vi "Dashboard Main.vi"() -> ()   [LabVIEW 2016]
uses:
  <vilib>/Rock Robotics/Network Tables/NT Read Numeric Array.vi
  <vilib>/Rock Robotics/Network Tables/NT Read Number.vi
  <vilib>/Rock Robotics/Network Tables/NT Write Number.vi
  <vilib>/Rock Robotics/Network Tables/NT Read Boolean.vi
panel:
  out "Camera Info":cluster{"Mbps LED":bool, "Mbps":dbl, "fps":dbl} {"fps" format="%#.1g"; "Mbps" format="%#.1g"}
  in  "Camera Settings":T1={"Frame Rate"=30, "Compression"=30, "Size"=1, "DB Camera Config"=FALSE} {"Frame Rate" scale=1.0..30.0; "Compression" scale=100.0..-1.0; "Size" items=["640x480", "320x240", "160x120"]}
  in  "TCP":refnum<k5>
  out "Robot IP":string
  in  "Dashboard Tab":T2(tab)
  in  "Select Auto":string(combo)
  out "NT Connection":bool
  out "MotorChart R":cluster{"Numeric":dbl, "Numeric":dbl}(graph)
  out "MotorChart L":cluster{"Numeric":dbl, "Numeric":dbl}(graph)
  out "MotorSliders R":cluster{"MotorSlide1":dbl, "MotorSlide2":dbl} {"MotorSlide2" scale=-1.0..1.0 scale format="%#_2e"; "MotorSlide1" scale=-1.0..1.0 scale format="%#_2e"}
  out "MotorSliders L":cluster{"MotorSlide1":dbl, "MotorSlide2":dbl} {"MotorSlide2" scale=-1.0..1.0 scale format="%#_2e"; "MotorSlide1" scale=-1.0..1.0 scale format="%#_2e"}
  out "JS1 Z":dbl(slide) scale=-1.0..1.0 scale format="%#_2e"
  out "JS1 Graph":cluster{"X":dbl, "Y":dbl}[](graph)
  out "JS1 Buttons":T3
  out "JS2 Z":dbl(slide) scale=-1.0..1.0 scale format="%#_2e"
  out "JS2 Graph":cluster{"X":dbl, "Y":dbl}[](graph)
  out "JS2 Buttons":T3
  out "Mode":T4(ring)=enum."Auto Disabled"
  in  "flywheelTarget":dbl
  out "Flywheel PID Graph":cluster{"Numeric":dbl, "Numeric":dbl}(graph)
  in  "flywheelF":dbl
  in  "flywheelD":dbl
  in  "flywheelI":dbl
  in  "flywheelP":dbl
  out "Drive PID Graph":cluster{"Numeric":dbl, "Numeric":dbl}(graph)
  in  "driveD":dbl
  in  "driveI":dbl
  in  "driveP":dbl
  out "gyroOnTarget":bool
  out "Gyro Exists":bool
  out "Gyro Heading PID":cluster{dbl, dbl}(knob) scale=-180.0..180.0
  in  "gyroD":dbl
  in  "gyroI":dbl
  in  "gyroP":dbl
  out "Tree":string(tree)
  out "Camera Image":T5(plugin-control)
  out "Background":bool
  in  "Camera Name":string(combo)="No Camera Selection"
  # "HW"
  # "Joysticks"
  # "Drive Motors"
  # "Front"
  # "Right"
  # "Left"
  # "Back"
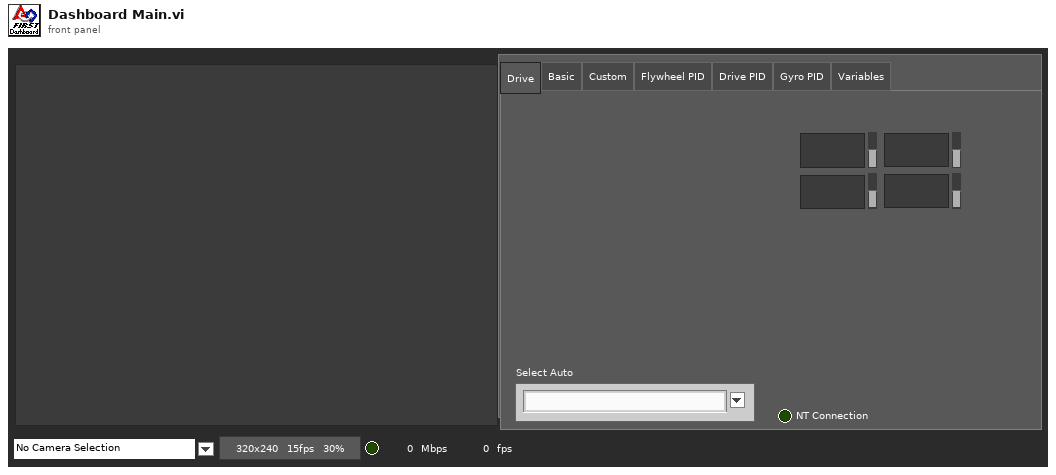
[diagram p1: front panel]
types:
  T1 = cluster{"Frame Rate":i32, "Compression":i32, "Size":u16, "DB Camera Config":bool}
  T2 = enum32{"Drive", "Basic", "Custom", "Flywheel PID", "Drive PID", "Gyro PID", "Variables"}
  T3 = cluster{bool, bool, bool, bool, bool, bool, bool, bool, bool, bool, bool, bool}
  T4 = enum8{"Tele-Op Disabled", "Tele-Op Enabled", "Auto Disabled", "Auto Enabled", "Test Disabled", "Test Enabled", "Disconnected", "No Code", "E-Stop"}
  T5 = typedef "IMAQ Image.ctl" = refnum<image>
  T6 = typedef "Image Type" = u32
  T7 = cluster{"Camera Image":refnum<vi>, "Dashboard Tab":refnum<vi>, "Background":refnum<vi>, "Tree":refnum<vi>, "Camera Settings":refnum<vi>, "Camera Name":refnum<vi>, "Camera Info":refnum<vi>}
  T8 = cluster{"Error Strings":string, "Disable Counts":cluster{u16, u16}, "Rail Faults":cluster{u16, u16, u16}, "Robot IP":string, "DB Mode":u8, "Event Info":cluster{"Name":string, "Type":u8, "Number":u16, "Replay":u8}}
  T9 = cluster{"Storage":cluster{"Disk Free":u64, "RAM Block":u32, "RAM free":u32}, "CPU Utilization":cluster{"CPU % ISR":sgl, "CPU % Time Crit":sgl, "CPU % Timed Str":sgl, "CPU % High":sgl, "CPU % Above":sgl, "CPU % Normal":sgl, "CPU % Low":sgl}, "CAN":cluster{"% Bus Utilization":sgl, "Bus Off Cnt":u32, "TX_FIFO Full Cnt":u32, "Receive Error Cnt":u8, "Transmit Error Cnt":u8}, "HID":cluster{"HID Outputs":u32, "Rumble Low":u16, "Rumble High":u16}[]}
  T10 = cluster{"Status bits":cluster{"Test Mode":bool, "Autonomous":bool, "Enabled":bool, "Code Start":bool, "Brownout":bool, "Reserved 2":bool, "Reserved 3":bool, "E-Stop":bool}, "Code Trace":cluster{"Disabled":bool, "TeleOp":bool, "Auto":bool, "Test":bool}, "Controller Type":enum16{"unknown", "cRIO", "roboRio"}, "Code?":enum16{"unknown", "noCode", "code"}, "Battery V":dbl}
  T11 = cluster{"Control Bits":cluster{"TestMode":bool, "Autonomous":bool, "Enabled":bool, "FMS Present":bool, bool, bool, bool, "E-Stop":bool}, "Team Station ":u8, "Countdown":sgl, "Joystick Values":cluster{"Axes":dbl[], "Buttons":bool[], "POVs":i16[]}[]}
  T12 = cluster{"Axes":dbl[], "Buttons":bool[], "POVs":i16[]}[]
  T13 = cluster{"Axes":dbl[], "Buttons":bool[], "POVs":i16[]}
  T14 = cluster{"Buttons[0]":bool, "Buttons[1]":bool, "Buttons[2]":bool, "Buttons[3]":bool, "Buttons[4]":bool, "Buttons[5]":bool, "Buttons[6]":bool, "Buttons[7]":bool, "Buttons[8]":bool, "Buttons[9]":bool, "Buttons[10]":bool, "Buttons[11]":bool}
  T15 = cluster{"Shift":bool, "Ctrl":bool, "Alt":bool, "Cmd":bool, "Opt":bool}
  T16 = typedef "WPI_DriverStationRobotMode2.ctl" = enum16{"Autonomous Disabled", "Autonomous Enabled", "Teleop Disabled", "Teleop Enabled", "Disconnected", "Finish", "Test Disabled", "Test Enabled", "Emergency Stopped"}
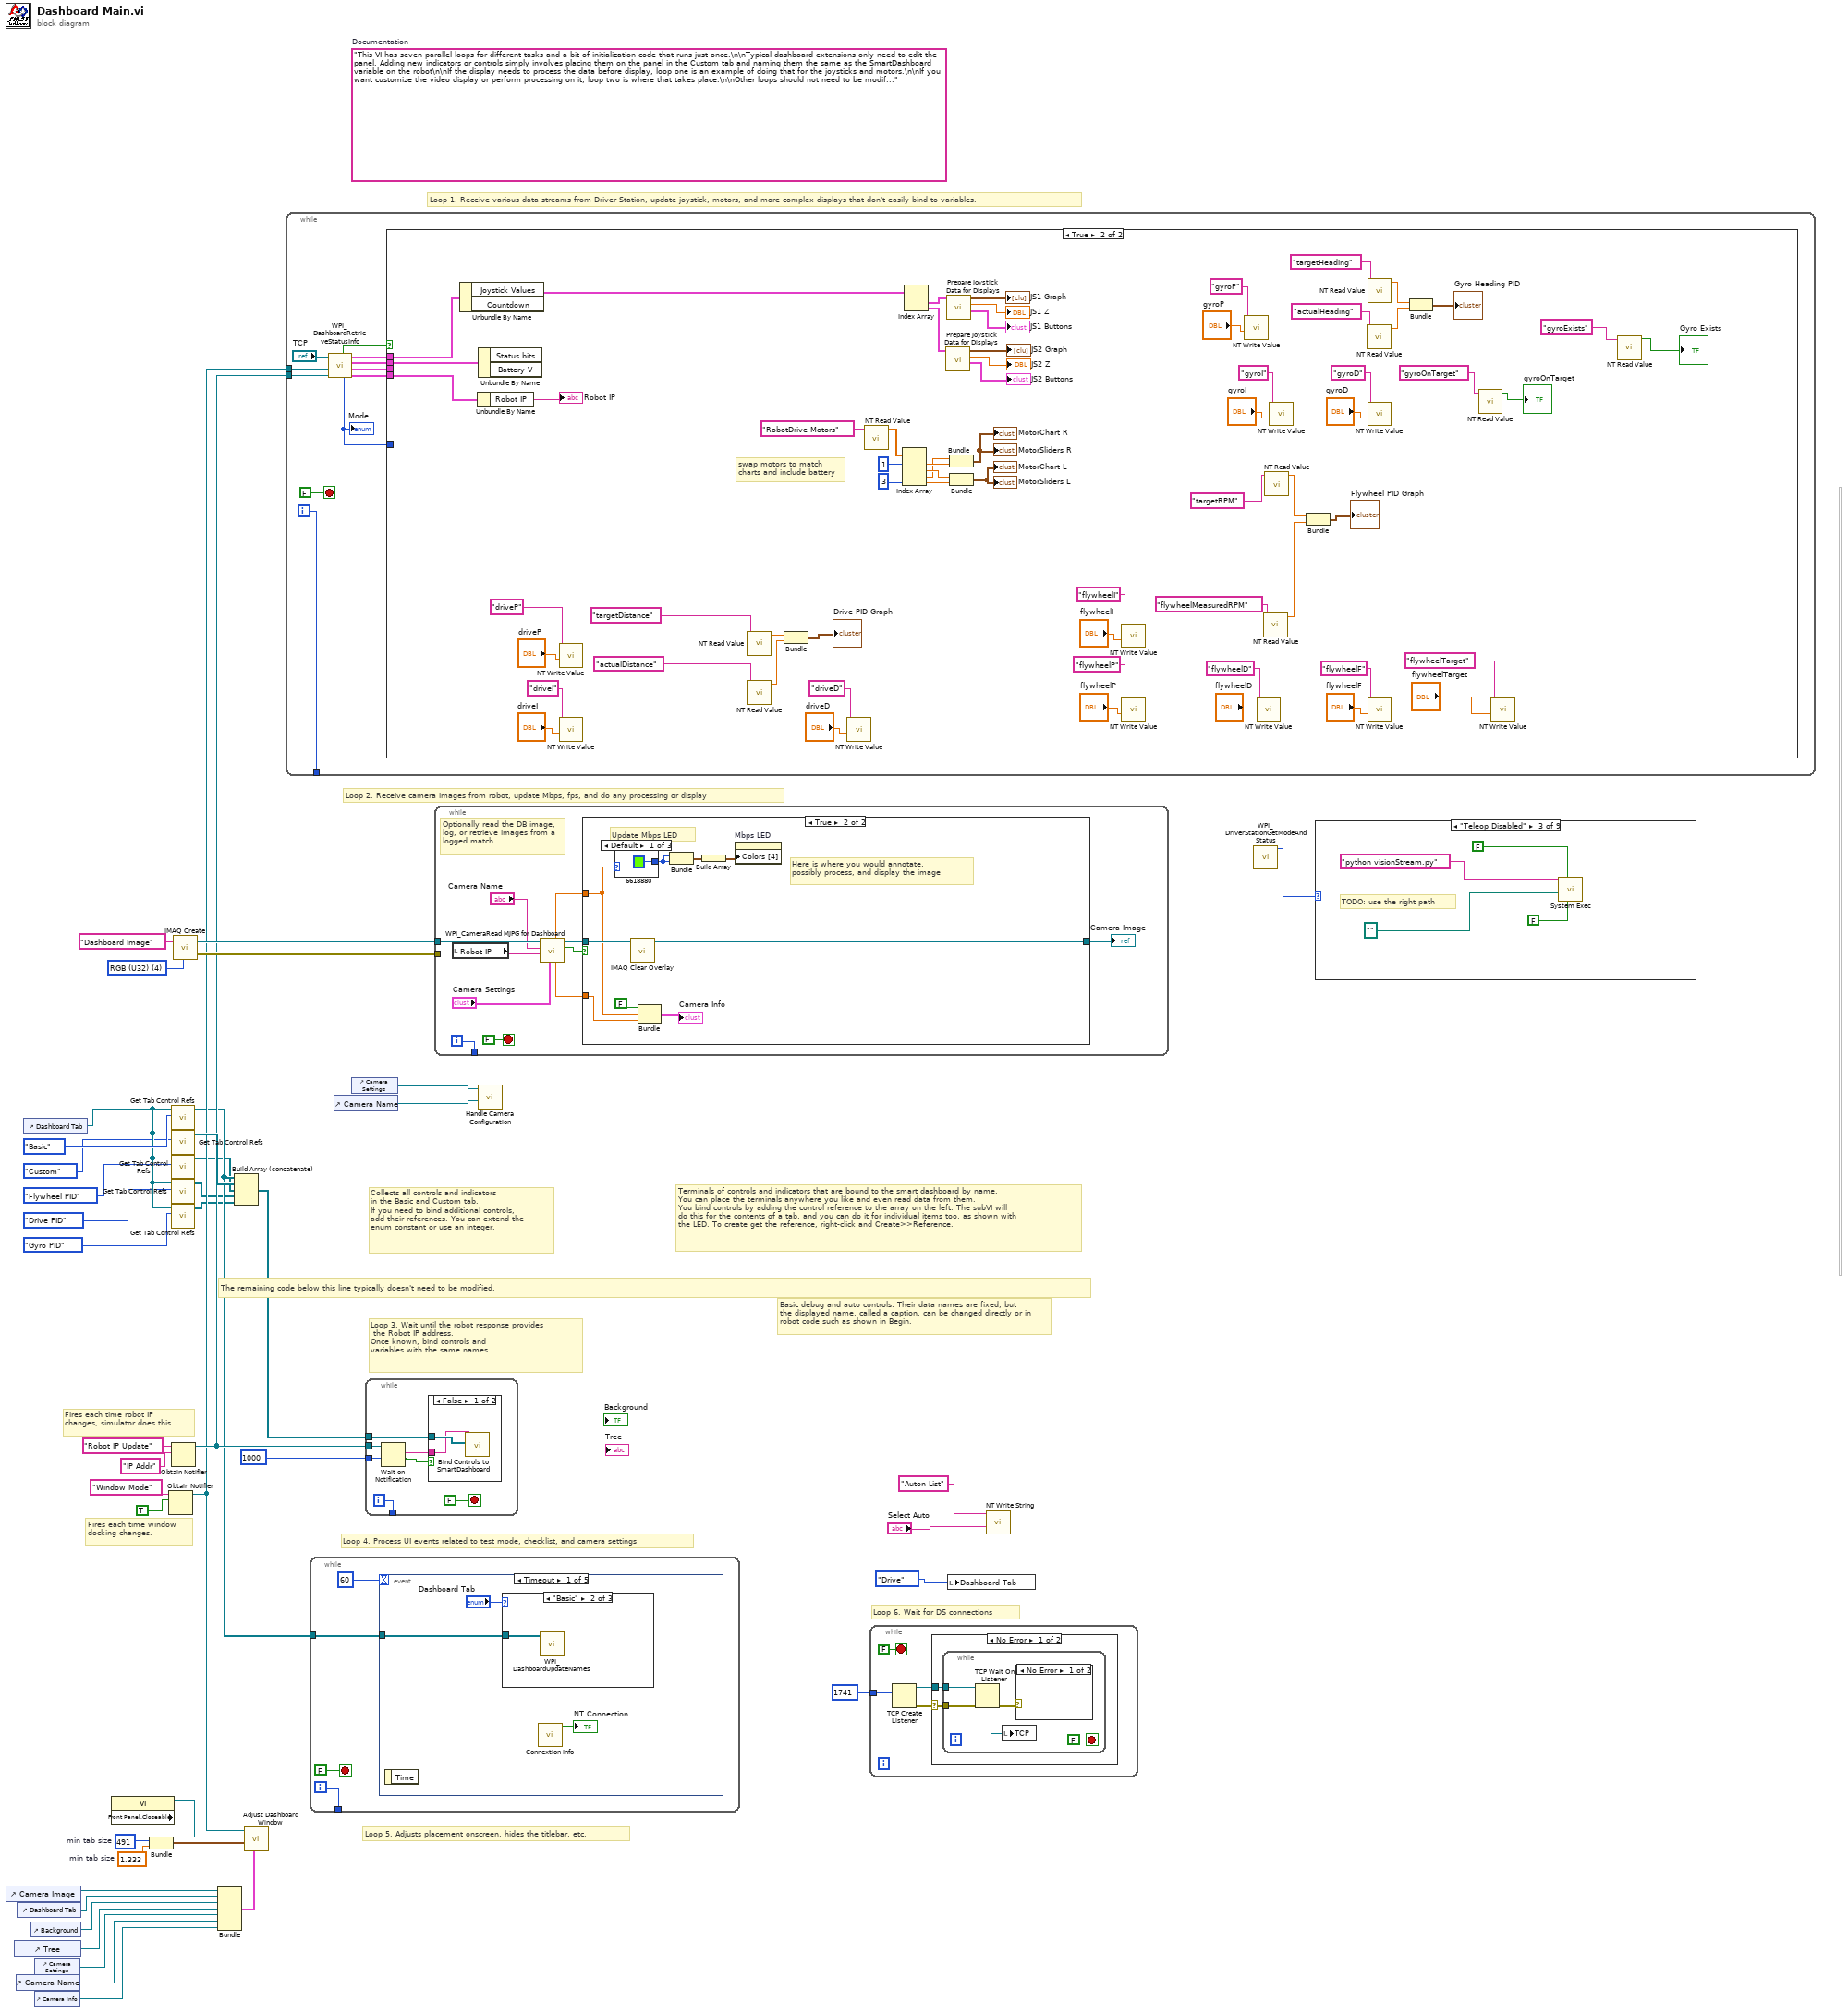
[diagram p0: block diagram]
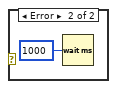
[diagram p10: hidden frame]
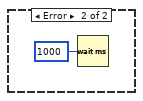
[diagram p11: hidden frame]
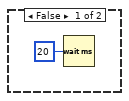
[diagram p12: hidden frame]
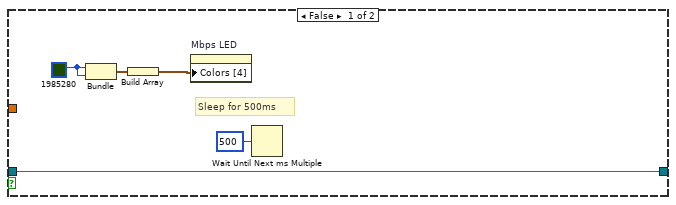
[diagram p14: hidden frame]
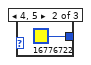
[diagram p15: hidden frame]
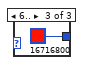
[diagram p16: hidden frame]
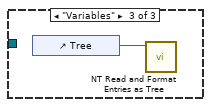
[diagram p18: hidden frame]
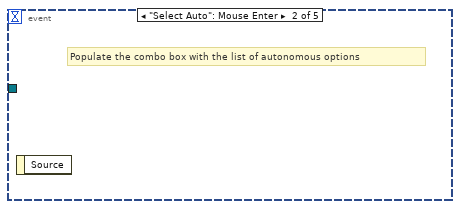
[diagram p19: hidden frame]
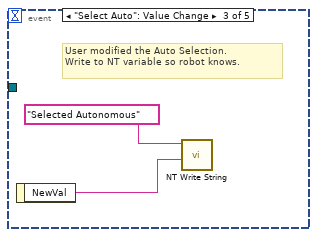
[diagram p20: hidden frame]
diagram:
  w28 = 491  # min tab size
  w27 = 1.333  # min tab size
  (unwired) "This VI has seven parallel loops for different tasks and a bit of initialization code that runs just once.\n\nTypical dashboard extensions only need to edit the panel. Adding new indicators or controls simply involves placing them on the panel in the Custom tab and naming them the same as the SmartDashboard variable on the robot\n\nIf the display needs to process the data before display, loop one is an example of doing that for the joysticks and motors.\n\nIf you want customize the video display or perform processing on it, loop two is where that takes place.\n\nOther loops should not need to be modified. They are pretty standard, and document the task they perform."  # Documentation
  w42 = T6 4 items=["Grayscale (U8)", "Grayscale (I16)", "Grayscale (SGL)", "Complex (CSG)", "RGB (U32)", "HSL (U32)", "RGB (U64)"] ("Image Type")
  # "Loop 6. Wait for DS connections"
  # "Basic debug and auto controls: Their data names are fixed, but\nthe displayed name, called a caption, can be changed directly or in\nrobot code such as shown in Begin."
  # "Fires each time robot IP\nchanges, simulator does this"
  # "Fires each time window\ndocking changes."
  # "Collects all controls and indicators\nin the Basic and Custom tab.\nIf you need to bind additional controls,\nadd their references. You can extend the\nenum constant or use an integer."
  # "The remaining code below this line typically doesn't need to be modified."
  # "Loop 4. Process UI events related to test mode, checklist, and camera settings"
  # "Terminals of controls and indicators that are bound to the smart dashboard by name.\nYou can place the terminals anywhere you like and even read data from them.\nYou bind controls by adding the control reference to the array on the left. The subVI will\ndo this for the contents of a tab, and you can do it for individual items too, as shown with\nthe LED. To create get the reference, right-click and Create>>Reference."
  # "Loop 3. Wait until the robot response provides\n the Robot IP address.\nOnce known, bind controls and\nvariables with the same names."
  # "Loop 5. Adjusts placement onscreen, hides the titlebar, etc."
  # "Loop 1. Receive various data streams from Driver Station, update joystick, motors, and more complex displays that don't easily bind to variables."
  # "Loop 2. Receive camera images from robot, update Mbps, fps, and do any processing or display"
  n1 = control-ref of="Camera Image"() -> (w30:refnum<vi>)
  n2 = control-ref of="Tree"() -> (w16:refnum<vi>)
  n3 = control-ref of="Camera Name"() -> (w14:refnum<vi>)
  n4 = control-ref of="Dashboard Tab"() -> (w29:refnum<vi>)
  n5 = control-ref of="Dashboard Tab"() -> (w8:refnum<vi>)
  n6 = control-ref of="Background"() -> (w25:refnum<vi>)
  n7 = control-ref of="Camera Settings"() -> (w15:refnum<vi>)
  n8 = control-ref of="Camera Info"() -> (w13:refnum<vi>)
  n9 = property class="VI" props=["Front Panel.Closeable"]() -> (reference out=w33:refnum<vi>)  [unwired: 2 in, 2 out]
  n10 = Bundle("min tab size"=w28, "min tab size"=w27) -> (w26:cluster{"min tab size":i32, "min tab size":dbl})  [unwired: 1 in]
  n11 = Obtain Notifier(name (unnamed)="Window Mode", notification data type=TRUE) -> (notifier out=w22:refnum<notifier>)  [unwired: 2 in, 2 out]
  n12 = call <vilib>:"Get Tab Control Refs.vi"("Page Index"=T2."Basic" ("Dashboard Tab"), "TabControl in"=w8) -> ("ControlsOnPage"=w18:refnum<vi>[])  [unwired: 9 in]
  n13 = call <vilib>:"Get Tab Control Refs.vi"("Page Index"=T2."Custom" ("Dashboard Tab"), "TabControl in"=w8) -> ("ControlsOnPage"=w32:refnum<vi>[])  [unwired: 9 in]
  n14 = call <vilib>:"Get Tab Control Refs.vi"("Page Index"=T2."Flywheel PID" ("Dashboard Tab"), "TabControl in"=w8) -> ("ControlsOnPage"=w10:refnum<vi>[])  [unwired: 9 in]
  n15 = call <vilib>:"Get Tab Control Refs.vi"("Page Index"=T2."Drive PID" ("Dashboard Tab"), "TabControl in"=w8) -> ("ControlsOnPage"=w3:refnum<vi>[])  [unwired: 9 in]
  n16 = call <vilib>:"Get Tab Control Refs.vi"("Page Index"=T2."Gyro PID" ("Dashboard Tab"), "TabControl in"=w8) -> ("ControlsOnPage"=w2:refnum<vi>[])  [unwired: 9 in]
  n17 = Obtain Notifier(name (unnamed)="Robot IP Update", notification data type="IP Addr" ("name (unnamed)")) -> (notifier out=w23:refnum<notifier>)  [unwired: 2 in, 2 out]
  n18 = call "IMAQ Create"("Image Name"="Dashboard Image", "Image Type"=w42) -> ("New Image"=w40:T5, "error out"=w39:errorcluster)  [unwired: 2 in, 1 out]
  n19 = Bundle("Camera Image"=w30, "Dashboard Tab"=w29, "Background"=w25, "Tree"=w16, "Camera Settings"=w15, "Camera Name"=w14, "Camera Info"=w13) -> (w24:T7)  [unwired: 1 in]
  n20 = Build Array (concatenate)(w18, w32, w10, w3, w2) -> (w31:refnum<vi>[])
  n21 = call "Adjust Dashboard Window.vi"("Sizing Refnums"=w24, "Size Constraints"=w26, "VI"=w33, "WIn Mode"=w22) -> ()  [unwired: 8 in]
  n22 = while {
    tunnel: [w52] -> _
    tunnel: w23 -> [w46]
    tunnel: w22 -> [w43]
    i -> [w52]
    stop <- FALSE stop-if-true
    n23 = call <vilib>:"WPI_DashboardRetrieveStatusInfo.vi"("Binding Refnum"=w46, "Window Mode Notifier"=w43, "TCP Cnx"="TCP") -> ("Power and Errors"=w47:T8, "Robot Metrics"=w50:T9, "Status Info"=w51:T10, "Control Info"=w48:T11, "Robot Mode"=w45:T4, "Process?"=w49:bool)  [unwired: 3 in]
    "Mode" <- w45
    n24 = case shown="True" w49 {
      tunnel: w51 -> [_ w117]
      tunnel: w50 -> [_ _]
      tunnel: w48 -> [_ w116]
      tunnel: w47 -> [_ w115]
      tunnel: w45 -> [_ _]
      frame False {
        n25 = Wait (ms)(milliseconds to wait=u32 20) -> ()  [unwired: 1 out]
      }
      frame True {
        # "swap motors to match\ncharts and include battery"
        n26 = Unbundle By Name(w116) -> ("Joystick Values"=w106:T12)  [unwired: 1 out]
        n27 = Unbundle By Name(w115) -> ("Robot IP"=→"Robot IP":string)
        n28 = Unbundle By Name(w117) -> ()  [unwired: 2 out]
        n29 = call-poly <vilib>:"NT Write Value.vi"("Numeric"="driveP", "Name"="driveP") -> ()  [unwired: 9 in, 1 out]
        n30 = call-poly <vilib>:"NT Write Value.vi"("Numeric"="driveI", "Name"="driveI") -> ()  [unwired: 9 in, 1 out]
        n31 = call-poly <vilib>:"NT Read Value.vi"("Name"="targetDistance") -> ("Numeric"=w58:dbl)  [unwired: 9 in, 1 out]
        n32 = call-poly <vilib>:"NT Read Value.vi"("Name"="actualDistance") -> ("Numeric"=w55:dbl)  [unwired: 9 in, 1 out]
        n33 = Bundle("Numeric"=w58, "Numeric"=w55) -> (→"Drive PID Graph":cluster{"Numeric":dbl, "Numeric":dbl})  [unwired: 1 in]
        n34 = call-poly <vilib>:"NT Write Value.vi"("Numeric"="driveD", "Name"="driveD") -> ()  [unwired: 9 in, 1 out]
        n35 = call-poly <vilib>:"NT Read Value.vi"("Name"="RobotDrive Motors") -> ("Numeric Array"=w96:dbl[])  [unwired: 9 in, 1 out]
        n36 = Index Array(array=w96, index #1=1, index #4=3) -> (element #1=w110:dbl, element #2=w111:dbl, element #3=w109:dbl, element #4=w114:dbl)  [unwired: 2 in]
        n37 = Index Array(array=w106) -> (element #1=w105:T13, element #2=w101:T13)  [unwired: 2 in]
        n38 = call "Prepare Joystick Data for Displays.vi"("Joystick Values"=w101) -> ("Buttons"=→"JS2 Buttons":T14, "Z Axis"=→"JS2 Z":dbl, "Cartesian Data"=→"JS2 Graph":cluster{"X axis":dbl, "X axis":dbl}[])  [unwired: 8 in]
        n39 = call "Prepare Joystick Data for Displays.vi"("Joystick Values"=w105) -> ("Buttons"=→"JS1 Buttons":T14, "Z Axis"=→"JS1 Z":dbl, "Cartesian Data"=→"JS1 Graph":cluster{"X axis":dbl, "X axis":dbl}[])  [unwired: 8 in]
        n40 = Bundle("Numeric"=w109, "Numeric"=w110) -> (→"MotorChart R" →"MotorSliders R":cluster{"Numeric":dbl, "Numeric":dbl})  [unwired: 1 in]
        n41 = Bundle("Numeric"=w111, "Numeric"=w114) -> (→"MotorChart L" →"MotorSliders L":cluster{"Numeric":dbl, "Numeric":dbl})  [unwired: 1 in]
        n42 = call-poly <vilib>:"NT Write Value.vi"("Numeric"="flywheelI", "Name"="flywheelI") -> ()  [unwired: 9 in, 1 out]
        n43 = call-poly <vilib>:"NT Write Value.vi"("Numeric"="flywheelP", "Name"="flywheelP") -> ()  [unwired: 9 in, 1 out]
        n44 = call-poly <vilib>:"NT Write Value.vi"("Numeric"="gyroP", "Name"="gyroP") -> ()  [unwired: 9 in, 1 out]
        n45 = call-poly <vilib>:"NT Write Value.vi"("Name"="flywheelD") -> ()  [unwired: 10 in, 1 out]
        n46 = call-poly <vilib>:"NT Read Value.vi"("Name"="flywheelMeasuredRPM") -> ("Numeric"=w80:dbl)  [unwired: 9 in, 1 out]
        n47 = call-poly <vilib>:"NT Read Value.vi"("Name"="targetRPM") -> ("Numeric"=w77:dbl)  [unwired: 9 in, 1 out]
        n48 = call-poly <vilib>:"NT Write Value.vi"("Numeric"="gyroI", "Name"="gyroI") -> ()  [unwired: 9 in, 1 out]
        n49 = Bundle("Numeric"=w77, "Numeric"=w80) -> (→"Flywheel PID Graph":cluster{"Numeric":dbl, "Numeric":dbl})  [unwired: 1 in]
        n50 = call-poly <vilib>:"NT Read Value.vi"("Name"="actualHeading") -> ("Numeric"=w87:dbl)  [unwired: 9 in, 1 out]
        n51 = call-poly <vilib>:"NT Read Value.vi"("Name"="targetHeading") -> ("Numeric"=w85:dbl)  [unwired: 9 in, 1 out]
        n52 = call-poly <vilib>:"NT Write Value.vi"("Numeric"="gyroD", "Name"="gyroD") -> ()  [unwired: 9 in, 1 out]
        n53 = call-poly <vilib>:"NT Write Value.vi"("Numeric"="flywheelF", "Name"="flywheelF") -> ()  [unwired: 9 in, 1 out]
        n54 = Bundle("Numeric"=w85, "Numeric"=w87) -> (→"Gyro Heading PID":cluster{"Numeric":dbl, "Numeric":dbl})  [unwired: 1 in]
        n55 = call-poly <vilib>:"NT Read Value.vi"("Name"="gyroOnTarget") -> ("Boolean"=→"gyroOnTarget":bool)  [unwired: 9 in, 1 out]
        n56 = call-poly <vilib>:"NT Write Value.vi"("Numeric"="flywheelTarget", "Name"="flywheelTarget") -> ()  [unwired: 9 in, 1 out]
        n57 = call-poly <vilib>:"NT Read Value.vi"("Name"="gyroExists") -> ("Boolean"=→"Gyro Exists":bool)  [unwired: 9 in, 1 out]
      }
    }
  }
  n58 = while {
    tunnel: [w119] -> _
    tunnel: w18 -> [w118]
    i -> [w119]
    stop <- FALSE stop-if-true
    n59 = event shown="[0] Timeout" {
      selector: _ -> [_ _ _ _ _]
      dyn-events: _ -> [_ _ _ _ _]
      timeout: u32 60 ("milliseconds to wait") -> [_ _ _ _ _]
      tunnel: w118 -> [w122 _ _ _ _]
      event Timeout {
        n60 = event-data() -> ()  [unwired: 1 in, 1 out]
        n61 = case shown="\"Basic\"" "Dashboard Tab" {
          tunnel: w122 -> [_ w125 _]
          frame "Custom", Default {
          }
          frame "Basic" {
            n62 = call <vilib>:"WPI_DashboardUpdateNames.vi"("Controls on Tab"=w125) -> ()  [unwired: 11 in]
          }
          frame "Variables" {
            n63 = control-ref of="Tree"() -> (w126:refnum<vi>)
            n64 = call <vilib>:"NT Read and Format Entries as Tree.vi"("Tree Refnum"=w126) -> ()  [unwired: 9 in, 2 out]
          }
        }
        n65 = call <vilib>:"Connextion Info.vi"() -> ("Connected"=→"NT Connection":bool)  [unwired: 10 in, 1 out]
      }
      event "Select Auto": Mouse Enter {
        # "Populate the combo box with the list of autonomous options"
        n66 = event-data() -> ()  [unwired: 1 in, 1 out]
      }
      event "Select Auto": Value Change {
        # "User modified the Auto Selection.\nWrite to NT variable so robot knows."
        n67 = event-data() -> ("NewVal"=w127:string)  [unwired: 1 in]
        n68 = call <vilib>:"NT Write String.vi"("String"=w127, "Name"="Selected Autonomous") -> ()  [unwired: 9 in, 1 out]
      }
      event Panel Close {
        n69 = event-data() -> ()  [unwired: 1 in, 1 out]
        n70 = invoke class="VI" method="Abort VI"() -> ()  [unwired: 3 in, 3 out]
      }
      event "Tree": Double Click {
        # "Update variable's persistence setting"
        n71 = event-data() -> ("PlatMods"=w132:T15, "Tag"=w131:string)  [unwired: 1 in]
        n72 = Unbundle(w132) -> ("Shift"=w130:bool)  [unwired: 4 out]
        n73 = Not(x=w130) -> (.not. x?=w129:bool)
        n74 = call <vilib>:"NT Update Persistence.vi"("Persistence"=w129, "Name"=w131) -> ()  [unwired: 9 in, 1 out]
      }
    }
  }
  n75 = control-ref of="Camera Name"() -> (w19:refnum<vi>)
  n76 = control-ref of="Camera Settings"() -> (w20:refnum<vi>)
  n77 = while {
    tunnel: w31 -> [w139]
    tunnel: w23 -> [w137]
    tunnel: [w135] -> _
    tunnel: u32 1000 ("milliseconds to wait") -> [w134]
    i -> [w135]
    stop <- FALSE stop-if-true
    n78 = Wait on Notification(notifier=w137, timeout in ms (-1)=w134) -> (notification=w136:string, timed out?=w133:bool)  [unwired: 2 in, 2 out]
    n79 = case shown="False" w133 {
      tunnel: w139 -> [w141 _]
      tunnel: w136 -> [w140 _]
      frame False {
        n80 = call <vilib>:"Bind Controls to SmartDashboard.vi"("Bound Control Refs"=w141, "Server IP Address"=w140) -> ()  [unwired: 10 in]
      }
      frame True {
      }
    }
  }
  n81 = while {
    tunnel: w40 -> [w150]
    tunnel: w39 -> [_]
    tunnel: [w151] -> _
    i -> [w151]
    stop <- FALSE stop-if-true
    # "Optionally read the DB image,\nlog, or retrieve images from a\nlogged match"
    n82 = local read "Robot IP"() -> (w146:string)
    n83 = call <vilib>:"WPI_CameraRead MJPG for Dashboard.vi"("Camera Settings"="Camera Settings", "Robot IP"=w146, "Camera Name"="Camera Name", "Refnum in"=w150) -> ("Active"=w148:bool, "Refnum out"=w149:T5, "FPS"=w147:dbl, "Bandwidth (Mbps)"=w145:dbl)  [unwired: 4 in]
    n84 = case shown="True" w148 {
      tunnel: w149 -> [w153 w164]
      tunnel: w145 -> [_ w161]
      tunnel: w147 -> [_ w162]
      tunnel: [w153 w158] -> w142
      frame False {
        w155 = u32 1985280 ("Color Box")
        # "Sleep for 500ms"
        n85 = Bundle("Color Box"=w155, "Color Box"=w155) -> (w156:cluster{"Color Box":u32, "Color Box":u32})  [unwired: 1 out]
        n86 = Build Array(w156) -> (w154:cluster{"Color Box":u32, "Color Box":u32}[])
        n87 = property on="Mbps LED" class="Bool (strict)"("Colors [4]"=w154) -> ()  [unwired: 2 in, 2 out]
        n88 = Wait Until Next ms Multiple(millisecond multiple=u32 500) -> ()  [unwired: 1 out]
      }
      frame True {
        # "Here is where you would annotate,\npossibly process, and display the image"
        # "Update Mbps LED"
        n89 = case shown="Default" w161 {
          tunnel: [u32 6618880 ("Color Box") u32 16776722 ("Color Box") u32 16716800 ("Color Box")] -> w165
          frame Default {
          }
          frame 4, 5 {
          }
          frame 6.. {
          }
        }
        n90 = call "IMAQ Clear Overlay"("Image"=w164) -> ("Image Out"=w158:T5)  [unwired: 2 in, 8 out]
        n91 = Bundle(FALSE, "Bandwidth (Mbps)"=w161, "FPS"=w162) -> (→"Camera Info":cluster{bool, "Bandwidth (Mbps)":dbl, "FPS":dbl})  [unwired: 1 in]
        n92 = Bundle("Color Box"=w165, "Color Box"=w165) -> (w166:cluster{"Color Box":u32, "Color Box":u32})  [unwired: 1 out]
        n93 = Build Array(w166) -> (w163:cluster{"Color Box":u32, "Color Box":u32}[])
        n94 = property on="Mbps LED" class="Bool (strict)"("Colors [4]"=w163) -> ()  [unwired: 2 in, 2 out]
      }
    }
    "Camera Image" <- w142
  }
  n95 = call "Handle Camera Configuration.vi"("CameraNameRef"=w19, "ClusterRef"=w20) -> ()  [unwired: 10 in]
  n96 = while {
    tunnel: u16 1741 ("timeout ms (25000)") -> [w171]
    stop <- FALSE stop-if-true
    n97 = TCP Create Listener(10:w171) -> (0:w170:errorcluster, 3:w172:refnum<k5>)  [unwired: 4 in, 1 out]
    n98 = case shown="No Error" w170 {
      selector: w170 -> [w174 _]
      tunnel: w172 -> [w175 _]
      frame No Error {
        n99 = while {
          tunnel: w175 -> [w178]
          tunnel: w174 -> [w177]
          stop <- FALSE stop-if-true
          n100 = TCP Wait On Listener(8:w177, 11:w178) -> (0:w179:errorcluster, 4:w180:refnum<k5>)  [unwired: 2 in, 3 out]
          n101 = local write "TCP"(w180) -> ()
          n102 = case shown="No Error" w179 {
            frame No Error {
            }
            frame Error {
              n103 = Wait (ms)(milliseconds to wait=u32 1000) -> ()  [unwired: 1 out]
            }
          }
        }
      }
      frame Error {
        n104 = Wait (ms)(milliseconds to wait=u32 1000) -> ()  [unwired: 1 out]
      }
    }
  }
  n105 = local write "Dashboard Tab"(T2."Drive" ("Dashboard Tab")) -> ()
  n106 = call <vilib>:"NT Write String.vi"("String"="Select Auto", "Name"="Auton List") -> ()  [unwired: 9 in, 1 out]
  n107 = call <vilib>:"WPI_DriverStationGetModeAndStatus.vi"() -> ("Robot Mode"=w1:T16)  [unwired: 10 in, 1 out]
  n108 = case shown="\"Teleop Disabled\"" w1 {
    frame "Autonomous Disabled", Default {
    }
    frame "Autonomous Enabled" {
    }
    frame "Teleop Disabled" {
      # "TODO: use the right path"
      n109 = call <vilib>:"System Exec.vi"("run minimized? (F)"=FALSE, "wait until completion? (T)"=FALSE, "working directory"=path "", "command line"="python visionStream.py") -> ()  [unwired: 4 in, 4 out]
    }
    frame "Teleop Enabled" {
    }
    frame "Disconnected" {
    }
    frame "Finish" {
    }
    frame "Test Disabled" {
    }
    frame "Test Enabled" {
    }
    frame "Emergency Stopped" {
    }
  }
